vi "Test.vi"(6 "stop":bool, 7 "Send":bool, 8 "error in (no error)":errorcluster, 9 "Relay No":i32, 10 "ON/OFF":bool, 11 "VISA resource name":refnum<visa-resource-name>) -> (0 "error out":errorcluster)   [LabVIEW 2023, in "Numato.lvlib"]
uses:
  Numato.lvlib
panel:
  in  "Open all":bool
  # "Starting from 1 instead of 0"
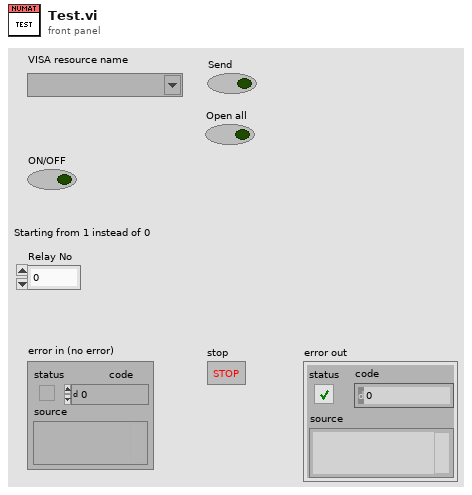
[diagram p1: front panel]
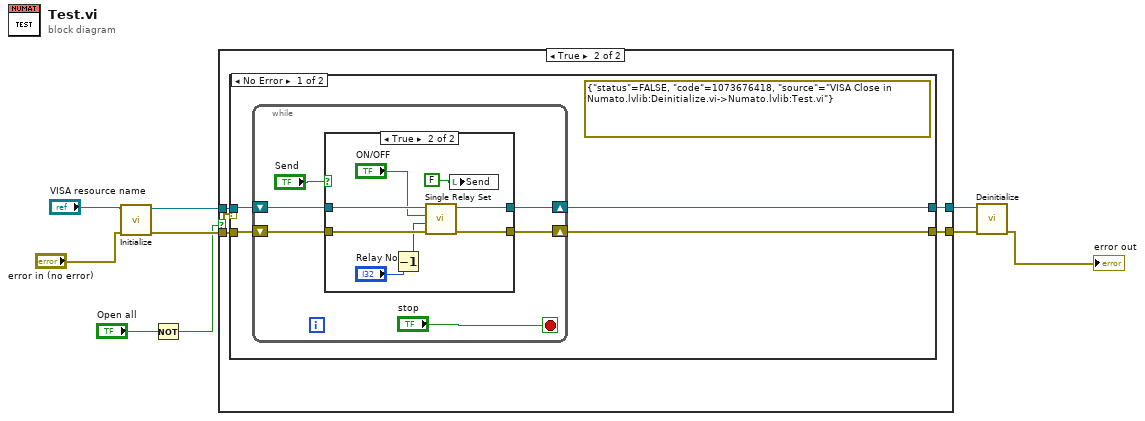
[diagram p0: block diagram]
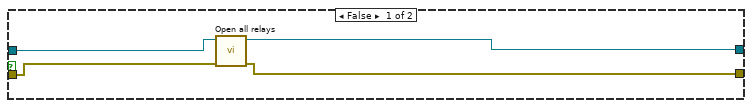
[diagram p2: hidden frame]
diagram:
  n1 = call "Initialize.vi"("error in (no error)"="error in (no error)", "Resource"="VISA resource name") -> ("error out"=w3:errorcluster, "VISA resource name out"=w7:refnum<visa-resource-name>)  [unwired: 8 in]
  n2 = Not(x="Open all") -> (.not. x?=w1:bool)
  n3 = case shown="True" w1 {
    tunnel: w7 -> [w13 w17]
    tunnel: [w10 w16] -> w6
    tunnel: [w11 w15] -> w5
    tunnel: w3 -> [w12 w14]
    frame False {
      n4 = call "Open all relays.vi"("error in (no error)"=w12, "VISA resource name"=w13) -> ("error out"=w11:errorcluster, "VISA resource name out"=w10:refnum<visa-resource-name>)  [unwired: 8 in]
    }
    frame True {
      n5 = case shown="No Error" w14 {
        tunnel: w17 -> [w21 w38]
        tunnel: [w20 w38] -> w16
        tunnel: w14 -> [w19 w39]
        tunnel: [w18 w39] -> w15
        frame No Error {
          (unwired) errorcluster {"status"=FALSE, "code"=1073676418, "source"="VISA Close in Numato.lvlib:Deinitialize.vi->Numato.lvlib:Test.vi"} ("error out 2")
          n6 = while {
            shift-right: [w26] -> w20
            shift-left: w21 -> [w27]
            shift-right: [w24] -> w18
            shift-left: w19 -> [w25]
            stop <- "stop" stop-if-true
            n7 = case shown="True" "Send" {
              tunnel: w27 -> [w29 w37]
              tunnel: [w29 w36] -> w26
              tunnel: w25 -> [w28 w35]
              tunnel: [w28 w34] -> w24
              frame False {
              }
              frame True {
                n8 = Decrement(x="Relay No") -> (x-1=w30:i32)
                n9 = call "Single Relay Set.vi"("error in (no error)"=w35, "Relay No"=w30, "ON/OFF"="ON/OFF", "VISA resource name"=w37) -> ("error out"=w34:errorcluster, "VISA resource name out"=w36:refnum<visa-resource-name>)  [unwired: 6 in]
                n10 = local write "Send"(FALSE ("Send")) -> ()
              }
            }
          }
        }
        frame Error {
        }
      }
    }
  }
  n11 = call "Deinitialize.vi"("error in (no error)"=w5, "VISA resource name"=w6) -> ("error out"=→"error out":errorcluster)  [unwired: 9 in]
